vi "Drive_CalculateMovement.vi"(3 "error in":errorcluster, 4 "Mode":T1, 5 "Y rel":dbl, 6 "X rel":dbl) -> (0 "error out":errorcluster, 2 "Movements":cluster{"Left":dbl, "Right":dbl}[](array[cluster]))   [LabVIEW 2009, in "Drive.lvlib"]
doc: "Calculates a sequence of movements to the specified point depending on the mode.\n\nFor TurnThenStraight mode outputs two movements - turning on spot then moving straight ahead."
uses:
  Drive.lvlib
  Drive_PositionControlMode.ctl
  Drive_Utils.lvlib
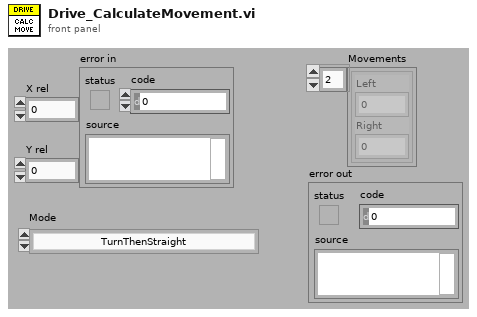
[diagram p1: front panel]
types:
  T1 = typedef "Drive.lvlib/Drive_PositionControlMode.ctl" = enum16{"TurnThenStraight"}
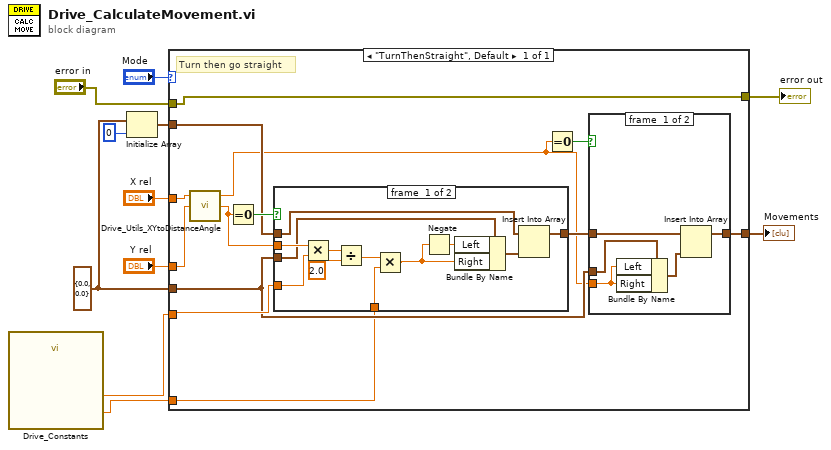
[diagram p0: block diagram]
diagram:
  w6 = cluster{"Left":dbl, "Right":dbl} {"Left"=0.0, "Right"=0.0} ("Movement")
  n1 = call "Drive_Constants.vi"() -> ("Wheels interval (m)"=w2:dbl, "Turning correction constant"=w1:dbl)  [unwired: 22 in, 4 out]
  n2 = Initialize Array(w6, 0 ("dimension size")) -> (w5:cluster{"Left":dbl, "Right":dbl}[])
  n3 = case shown="\"TurnThenStraight\", Default" "Mode" {
    tunnel: "X rel" -> [w24]
    tunnel: "Y rel" -> [w23]
    tunnel: w2 -> [w22]
    tunnel: [w15] -> w8
    tunnel: w6 -> [w19]
    tunnel: w5 -> [w18]
    tunnel: "error in" -> [w13]
    tunnel: [w13] -> w3
    tunnel: w1 -> [w12]
    frame "TurnThenStraight", Default {
      # "Turn then go straight"
      n4 = call "Drive_Utils_XYtoDistanceAngle.vi"("Y"=w23, "X"=w24) -> ("Angle (rad)"=w20:dbl, "Distance"=w14:dbl)  [unwired: 1 in, 1 out]
      n5 = Equal To 0?(x=w20) -> (x = 0?=w21:bool)
      n6 = case shown="False" w21 {
        tunnel: w20 -> [w42 _]
        tunnel: w22 -> [w41 _]
        tunnel: w19 -> [w37 _]
        tunnel: [w36 w43] -> w16
        tunnel: w18 -> [w34 w43]
        tunnel: w12 -> [w31 _]
        frame #0 {
          n7 = Multiply(x=w42, y=w41) -> (x*y=w40:dbl)
          n8 = Divide(x=w40, y=2.0) -> (x/y=w32:dbl)
          n9 = Multiply(x=w32, y=w31) -> (x*y=w33:dbl)
          n10 = Negate(x=w33) -> (-x=w38:dbl)
          n11 = Bundle By Name(cluster=w37, "Left"=w38, "Right"=w33) -> (w35:cluster{"Left":dbl, "Right":dbl})
          n12 = Insert Into Array(array=w34, new element=w35) -> (w36:cluster{"Left":dbl, "Right":dbl}[])  [unwired: 1 in]
        }
        frame #1 {
        }
      }
      n13 = Equal To 0?(x=w14) -> (x = 0?=w17:bool)
      n14 = case shown="False" w17 {
        tunnel: w19 -> [w29 _]
        tunnel: w14 -> [w28 _]
        tunnel: w16 -> [w27 w30]
        tunnel: [w26 w30] -> w15
        frame #0 {
          n15 = Bundle By Name(cluster=w29, "Left"=w28, "Right"=w28) -> (w25:cluster{"Left":dbl, "Right":dbl})
          n16 = Insert Into Array(array=w27, new element=w25) -> (w26:cluster{"Left":dbl, "Right":dbl}[])  [unwired: 1 in]
        }
        frame #1 {
        }
      }
    }
  }
  "Movements" <- w8
  "error out" <- w3
